vi "sv_Decimation by 2 with IC.vi"(2 "init/cont (init:F)":bool, 3 "initial decimation state":i32, 4 "X":dbl[](array[numeric]) format="%.2f") -> (0 "final decimation state":i32, 1 "decimated X":dbl[](array[numeric]) format="%.2f")   [LabVIEW 2017, in "SoundVib_Octave_2014 standard.lvlib"]
doc: "Decimates the X input array by 2.\n\nThe Initial Decimation State and Final Decimation State keep track of the internal state of the decimation process to insure continuous operation (if continuous mode is used)."
uses:
  <vilib>/addons/Sound and Vibration/svt_Octave/SoundVib_Octave_2014 standard.lvlib
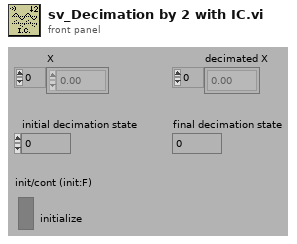
[diagram p1: front panel]
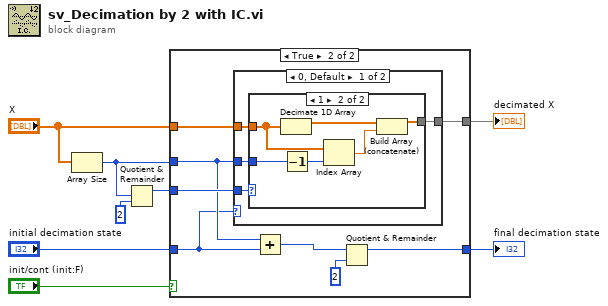
[diagram p0: block diagram]
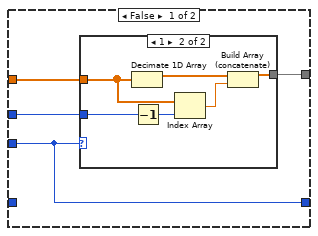
[diagram p2: hidden frame]
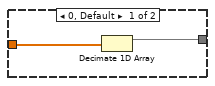
[diagram p3: hidden frame]
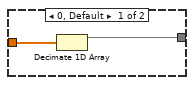
[diagram p4: hidden frame]
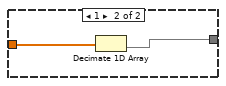
[diagram p5: hidden frame]
diagram:
  n1 = Array Size(array="X") -> (size(s)=w8:i32)
  n2 = Quotient & Remainder(x=w8, y=2) -> (x-y*floor(x/y)=w7:i32)  [unwired: 1 out]
  n3 = case shown="True" "init/cont (init:F)" {
    tunnel: "X" -> [w12 w25]
    tunnel: [w11 w24] -> w3
    tunnel: w8 -> [w10 w22]
    tunnel: [w9 w26] -> w4
    tunnel: "initial decimation state" -> [_ w21]
    tunnel: w7 -> [w9 w23]
    frame False {
      n4 = case shown="1" w9 {
        tunnel: w12 -> [w14 w17]
        tunnel: [w13 w15] -> w11
        tunnel: w10 -> [_ w16]
        frame 0, Default {
          n5 = Decimate 1D Array(w14) -> (w13:dbl[])  [unwired: 1 out]
        }
        frame 1 {
          n6 = Decimate 1D Array(w17) -> (w19:dbl[])  [unwired: 1 out]
          n7 = Decrement(x=w16) -> (x-1=w18:i32)
          n8 = Index Array(array=w17, index=w18) -> (element=w20:dbl)
          n9 = Build Array (concatenate)(w19, w20) -> (w15:dbl[])
        }
      }
    }
    frame True {
      n10 = case shown="0, Default" w21 {
        tunnel: w25 -> [w32 w42]
        tunnel: [w31 w41] -> w24
        tunnel: w22 -> [w30 _]
        tunnel: w23 -> [w29 _]
        frame 0, Default {
          n11 = case shown="1" w29 {
            tunnel: w32 -> [w34 w37]
            tunnel: [w33 w36] -> w31
            tunnel: w30 -> [_ w35]
            frame 0, Default {
              n12 = Decimate 1D Array(w34) -> (w33:dbl[])  [unwired: 1 out]
            }
            frame 1 {
              n13 = Decimate 1D Array(w37) -> (w39:dbl[])  [unwired: 1 out]
              n14 = Decrement(x=w35) -> (x-1=w38:i32)
              n15 = Index Array(array=w37, index=w38) -> (element=w40:dbl)
              n16 = Build Array (concatenate)(w39, w40) -> (w36:dbl[])
            }
          }
        }
        frame 1 {
          n17 = Decimate 1D Array(w42) -> (w41:dbl[])  [unwired: 1 out]
        }
      }
      n18 = Add(x=w22, y=w21) -> (x+y=w27:i32)
      n19 = Quotient & Remainder(x=w27, y=2) -> (x-y*floor(x/y)=w26:i32)  [unwired: 1 out]
    }
  }
  "final decimation state" <- w4
  "decimated X" <- w3
